vi "Motion_Convert Register to Double.vi"(7 "Start index":i32, 8 "Register array":u16[](array[numeric])) -> (2 "Double Value":dbl)   [LabVIEW 2010]
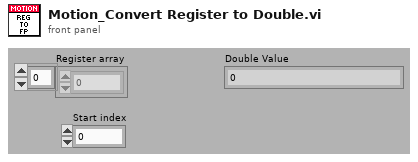
[diagram p1: front panel]
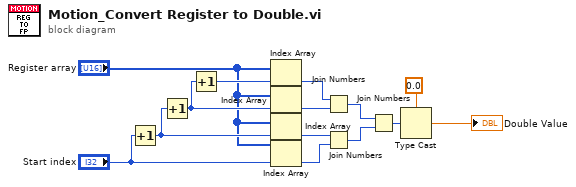
[diagram p0: block diagram]
diagram:
  n1 = Increment(x="Start index") -> (x+1=w3:i32)
  n2 = Increment(x=w3) -> (x+1=w4:i32)
  n3 = Increment(x=w4) -> (x+1=w5:i32)
  n4 = Index Array(array="Register array", index=w5) -> (element=w14:u16)
  n5 = Index Array(array="Register array", index=w4) -> (element=w13:u16)
  n6 = Index Array(array="Register array", index=w3) -> (element=w12:u16)
  n7 = Index Array(array="Register array", index="Start index") -> (element=w11:u16)
  n8 = Join Numbers(hi=w14, lo=w13) -> ((hi.lo)=w9:u32)
  n9 = Join Numbers(hi=w12, lo=w11) -> ((hi.lo)=w10:u32)
  n10 = Join Numbers(hi=w9, lo=w10) -> ((hi.lo)=w7:u64)
  n11 = Type Cast(type=0.0, x=w7) -> (*(type *) &x=→"Double Value":dbl)
